vi "lineare_tratti(subVi).vi"(7 "error in (no error)":errorcluster, 10 "Input":T1(plugin-control)) -> (0 "error out":errorcluster, 3 "New Image":T1)   [LabVIEW 2020]
uses:
  <vilib>/vision/Image Controls.llb/IMAQ Image.ctl
  <vilib>/vision/NI_Vision_Development_Module.lvlib
panel:
  out "Lookup Table":i32[](array[numeric])
  in  "stop":bool
  in  "m_B":sgl
  in  "X_B":u8
  in  "m_A":sgl
  in  "X_A":u8
  out "Trasformazione lineare a tratti":i32[](graph)
  out "OUTPUT":T1(plugin-control)
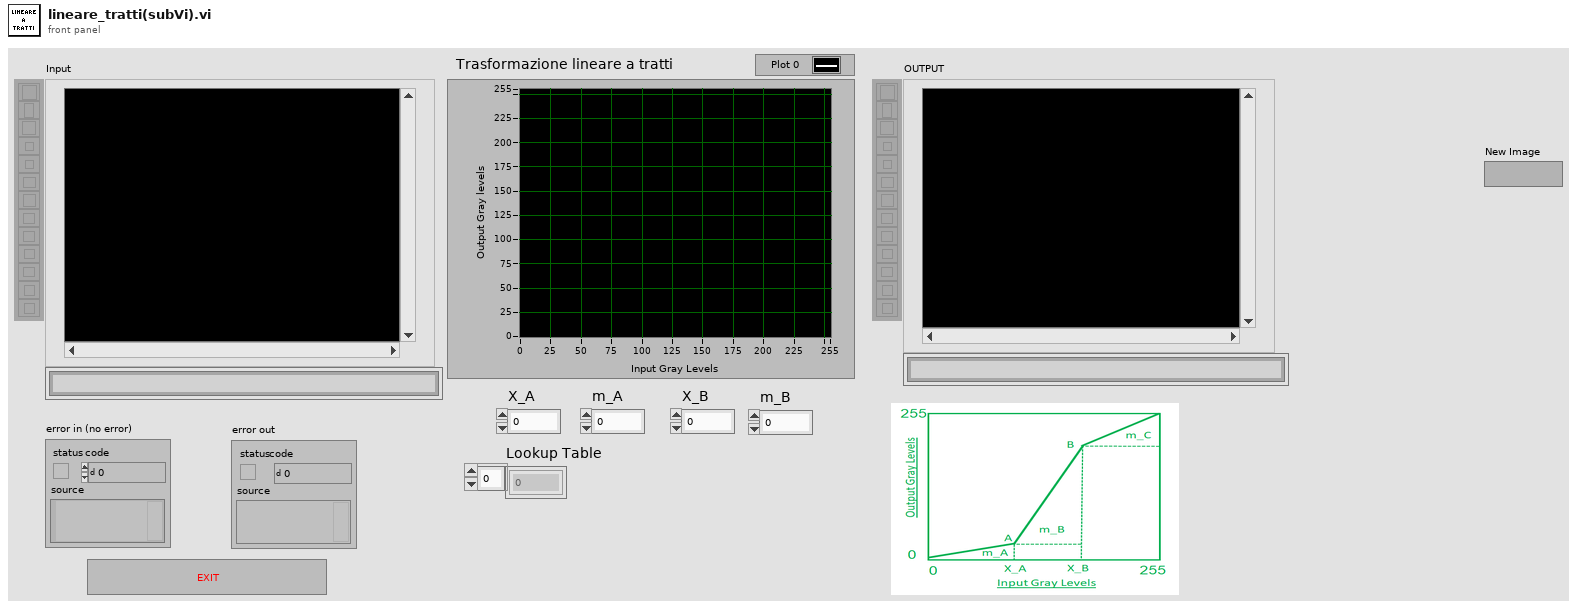
[diagram p1: front panel]
types:
  T1 = typedef "IMAQ Image.ctl" = refnum<image>
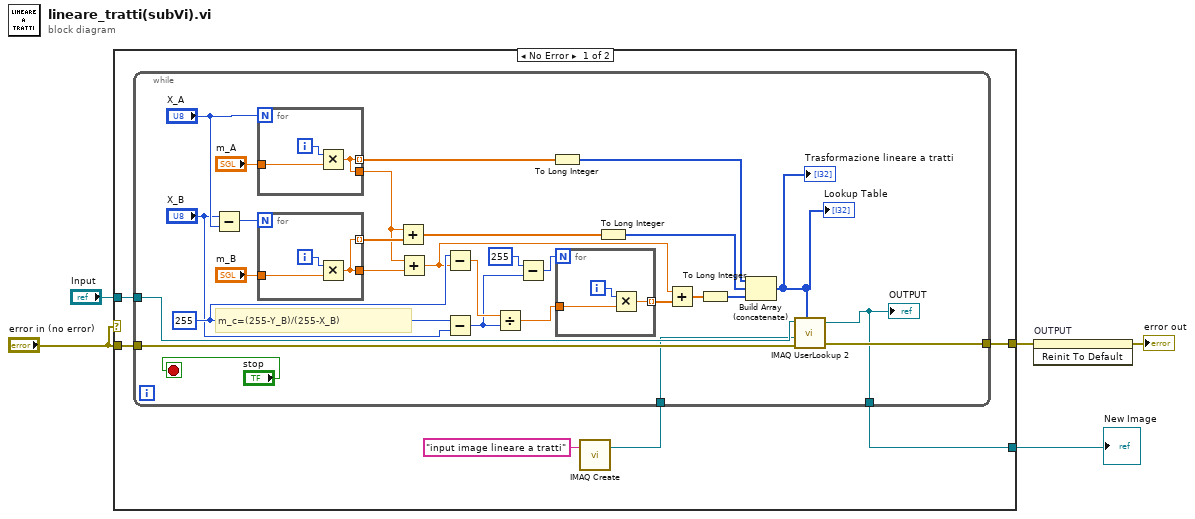
[diagram p0: block diagram]
diagram:
  n1 = case shown="No Error" "error in (no error)" {
    tunnel: [w11 w51] -> w5
    tunnel: "error in (no error)" -> [w10 w51]
    tunnel: "Input" -> [w9 w50]
    tunnel: [w6 w50] -> w1
    frame No Error {
      n2 = call "IMAQ Create"("Image Name"="input image lineare a tratti") -> ("New Image"=w7:T1)  [unwired: 4 in, 1 out]
      n3 = while {
        tunnel: [w18] -> w11
        tunnel: w10 -> [w17]
        tunnel: w9 -> [w16]
        tunnel: w7 -> [w13]
        tunnel: [w12] -> w6
        stop <- "stop" stop-if-true
        w32 = 255
        # "m_c=(255-Y_B)/(255-X_B)"
        n4 = Subtract(x="X_B", y="X_A") -> (x-y=w35:u8)
        n5 = for {
          N: "X_A" -> [_]
          tunnel: "m_A" -> [w48]
          tunnel: [w47] -> w40 mode=indexing
          tunnel: [w47] -> w33
          i -> [w49]
          n6 = Multiply(x=w49, y=w48) -> (x*y=w47:sgl)
        }
        n7 = for {
          N: w35 -> [_]
          tunnel: "m_B" -> [w46]
          tunnel: [w44] -> w38 mode=indexing
          tunnel: [w44] -> w34
          i -> [w45]
          n8 = Multiply(x=w45, y=w46) -> (x*y=w44:sgl)
        }
        n9 = Add(x=w33, y=w38) -> (x+y=w37:sgl[])
        n10 = Add(x=w33, y=w34) -> (x+y=w29:sgl)
        n11 = Subtract(x=w32, y=w29) -> (x-y=w31:sgl)
        n12 = Subtract(x=w32, y="X_B") -> (x-y=w24:i32)
        n13 = Divide(x=w31, y=w24) -> (x/y=w30:sgl)
        n14 = Subtract(x=u8 255, y=w24) -> (x-y=w23:i32)
        n15 = To Long Integer(number=w40) -> (32bit integer=w39:i32[])
        n16 = for {
          N: w23 -> [_]
          tunnel: w30 -> [w42]
          tunnel: [w41] -> w28 mode=indexing
          i -> [w43]
          n17 = Multiply(x=w43, y=w42) -> (x*y=w41:sgl)
        }
        n18 = To Long Integer(number=w37) -> (32bit integer=w36:i32[])
        n19 = Add(x=w29, y=w28) -> (x+y=w27:sgl[])
        n20 = To Long Integer(number=w27) -> (32bit integer=w26:i32[])
        n21 = Build Array (concatenate)(w39, w36, w26) -> (w15:i32[])
        "Trasformazione lineare a tratti" <- w15
        "Lookup Table" <- w15
        n22 = call "IMAQ UserLookup 2"("Image Src"=w16, "Lookup Table"=w15, "Image Dst"=w13, "error in (no error)"=w17) -> ("Image Dst Out"=w12:T1, "error out"=w18:errorcluster)  [unwired: 3 in]
        "OUTPUT" <- w12
      }
    }
    frame Error {
    }
  }
  "New Image" <- w1
  n23 = invoke on="OUTPUT" class="ImageControl" method="Reinit To Default"(error in=w5) -> (error out=→"error out":errorcluster)  [unwired: 2 in, 2 out]
